vi "Polynomial_convert.vi"(3 "Calib constants":dbl[](array[numeric])=[0.2727, 22.328, 22.281, -22.056, 13.889] format="%.3e", 6 "Voltage":dbl format="%.3f") -> (1 "Eng Values":dbl format="%.2f")   [LabVIEW 2010]
panel:
  # "x^0\nx^1\nx^2\nx^3\nx^4"
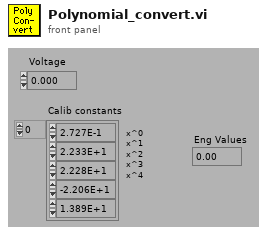
[diagram p1: front panel]
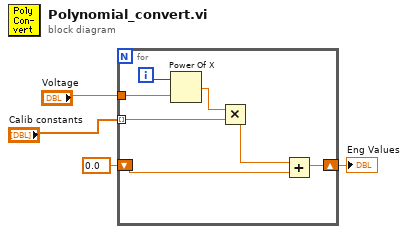
[diagram p0: block diagram]
diagram:
  n1 = for {
    shift-right: [w5] -> w2
    shift-left: 0.0 -> [w6]
    tunnel: "Voltage" -> [w10]
    tunnel: "Calib constants" -> [w8] mode=indexing
    i -> [w11]
    n2 = Power Of X(1:w10, 2:w11) -> (0:w9:dbl)
    n3 = Multiply(x=w9, y=w8) -> (x*y=w7:dbl)
    n4 = Add(x=w7, y=w6) -> (x+y=w5:dbl)
  }
  "Eng Values" <- w2
